vi "Read_All_Motor_Velocities.vi"(8 "Motor order":i32[](array[numeric]), 10 "error in (no error)":errorcluster, 11 "CanOpenConnectionsAllEposMotorDrivers":refnum<class "sbCANopenBaseClass.lvclass">[](array[class])) -> (2 "Motor velocities":i32[](array[numeric]), 3 "Motor position current velocity in columns":i32[][](array[numeric]))   [LabVIEW 2024]
uses:
  <vilib>/addons/Maxon Motor/EPOS2 CANopen/CANopen/sbCANopenBaseClass.lvclass
  <vilib>/addons/Maxon Motor/EPOS2 CANopen/EPOS2 Support Files/Typedefs/EPOS2 Data Output Current.ctl
  <vilib>/addons/Maxon Motor/EPOS2 CANopen/EPOS2 Support Files/Polymorphic SubVIs/Read PDO/EPOS2 Current Mode Read.vi
  <vilib>/addons/Maxon Motor/EPOS2 CANopen/EPOS2 Library.lvlib
panel:
  out "Data Output":T1
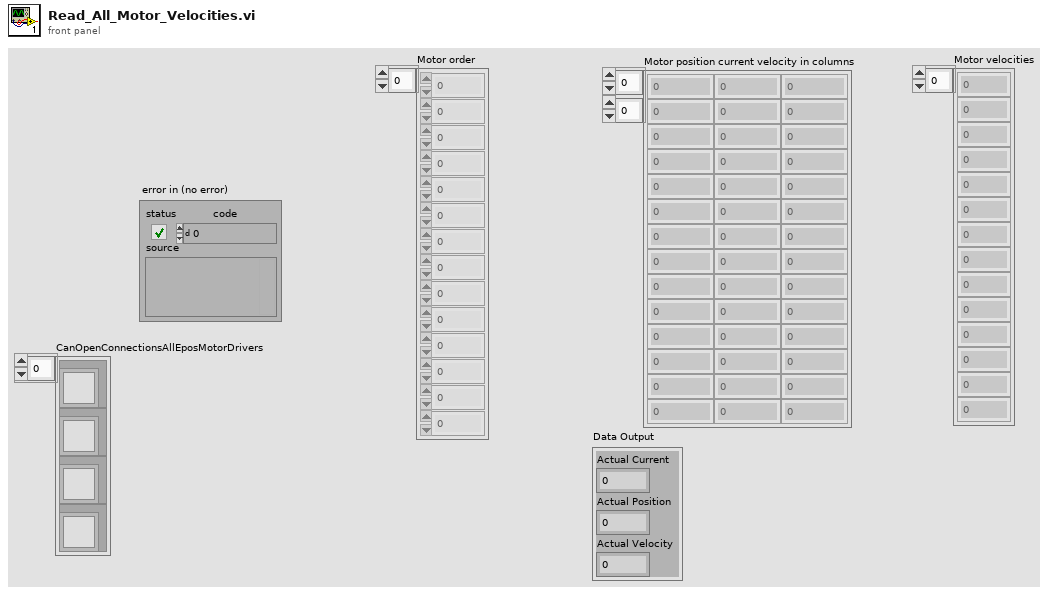
[diagram p1: front panel]
types:
  T1 = typedef "EPOS2 Library.lvlib/EPOS2 Data Output Current.ctl" = cluster{"Actual Current":i16, "Actual Position":i32, "Actual Velocity":i32}
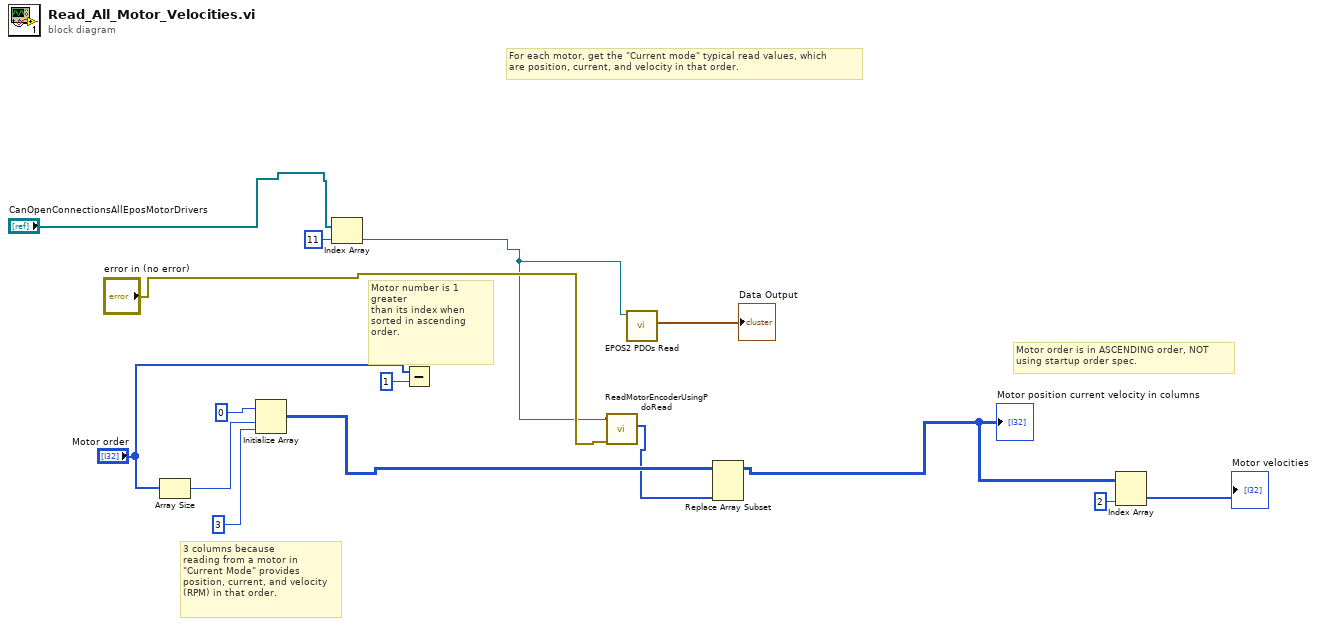
[diagram p0: block diagram]
diagram:
  # "Motor number is 1 greater\nthan its index when sorted in ascending\norder."
  # "3 columns because \nreading from a motor in \n\"Current Mode\" provides\nposition, current, and velocity\n(RPM) in that order."
  # "Motor order is in ASCENDING order, NOT\nusing startup order spec."
  # "For each motor, get the \"Current mode\" typical read values, which \nare position, current, and velocity in that order."
  n1 = Array Size(array="Motor order") -> (size(s)=w11:i32)
  n2 = Initialize Array(0 ("element"), w11, 3 ("dimension size")) -> (w10:i32[][])
  n3 = Index Array(array="CanOpenConnectionsAllEposMotorDrivers", index=11) -> (element=w2:refnum<class "sbCANopenBaseClass.lvclass">)
  n4 = Subtract(x="Motor order", y=1) -> ()  [unwired: 1 out]
  n5 = call "ReadMotorEncoderUsingPdoRead.vi"("error in (no error)"="error in (no error)", "CANopen Session In"=w2) -> ("ReadValues"=w5:i32[])  [unwired: 9 in]
  n6 = call-poly <vilib>:"EPOS2 PDOs Read.vi"("CANopen Session In"=w2) -> ("Data Output"=→"Data Output":T1)  [unwired: 7 in, 3 out]
  n7 = Replace Array Subset(array=w10, new element=w5) -> (w7:i32[][])  [unwired: 2 in]
  "Motor position current velocity in columns" <- w7
  n8 = Index Array(array=w7, index (col)=2 ("disabled index (col)")) -> (element=→"Motor velocities":i32[])  [unwired: 1 in]
